vi "sandbox.vi"() -> ()   [LabVIEW 2016]
panel:
  out "Array":i32[](array[numeric])
  out "RESET":bool
  out "ADDR (7bit)":u8
  out "R (U8)":u8
  out "G (U8)":u8
  out "B (U8)":u8
  in  "RESET":bool
  in  "ADDR (7bit)":u8
  in  "B (U8)":u8
  in  "G (U8)":u8
  out "Packet":u32=8 format="%032b"
  in  "R (U8)":u8
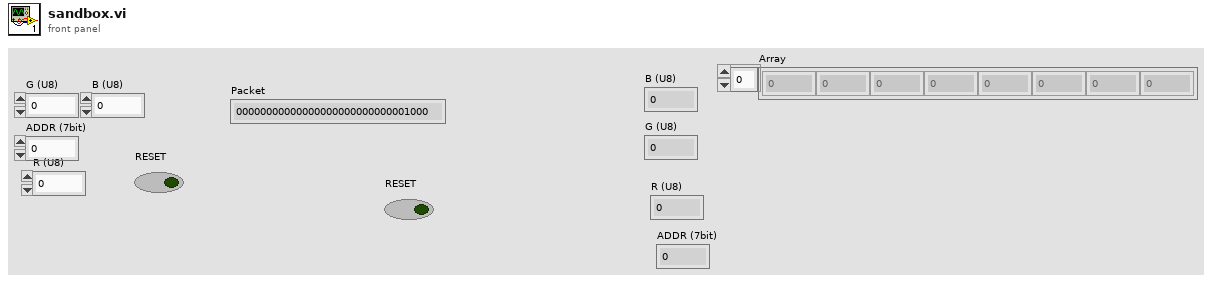
[diagram p1: front panel]
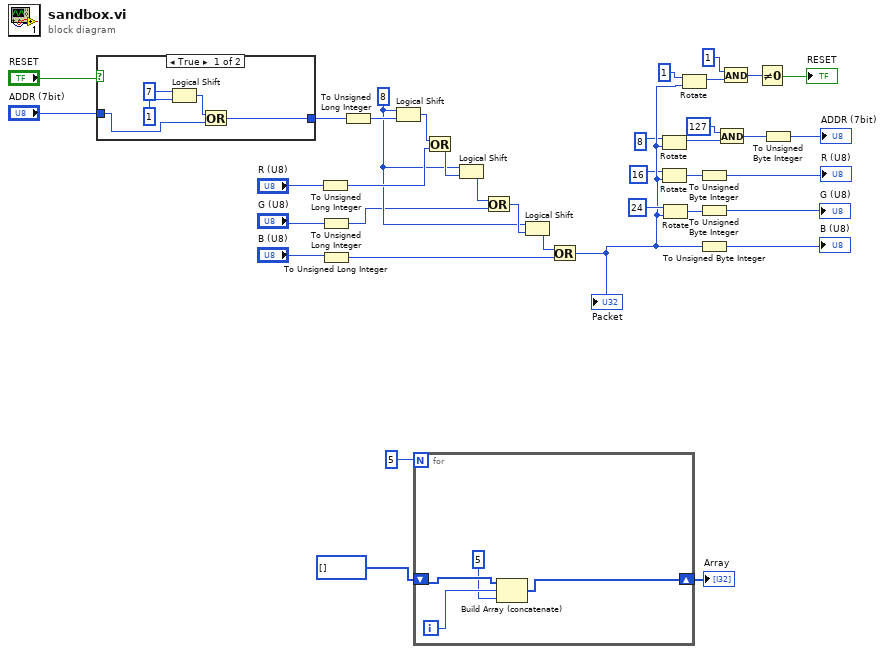
[diagram p0: block diagram]
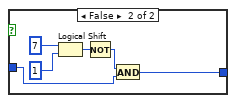
[diagram p2: hidden frame]
diagram:
  w26 = u8 8 ("x")
  n1 = case shown="True" "RESET" {
    tunnel: "ADDR (7bit)" -> [w39 w46]
    tunnel: [w38 w45] -> w33
    frame True {
      n2 = Logical Shift(y=u32 7, x=u8 1) -> (x << y=w40:u8)
      n3 = Or(x=w40, y=w39) -> (x .or. y?=w38:u8)
    }
    frame False {
      n4 = Logical Shift(y=u32 7, x=u8 1) -> (x << y=w47:u8)
      n5 = Not(x=w47) -> (.not. x?=w43:u8)
      n6 = And(x=w43, y=w46) -> (x .and. y?=w45:u8)
    }
  }
  n7 = To Unsigned Long Integer(number="R (U8)") -> (unsigned 32bit integer=w30:u32)
  n8 = To Unsigned Long Integer(number="G (U8)") -> (unsigned 32bit integer=w24:u32)
  n9 = To Unsigned Long Integer(number="B (U8)") -> (unsigned 32bit integer=w22:u32)
  n10 = To Unsigned Long Integer(number=w33) -> (unsigned 32bit integer=w32:u32)
  n11 = Logical Shift(y=w26, x=w32) -> (x << y=w31:u32)
  n12 = for {
    N: 5 ("Numeric") -> [_]
    shift-right: [w49] -> w2
    shift-left: i32[] [] -> [w52]
    i -> [w51]
    n13 = Build Array (concatenate)(w52, w51, 5) -> (w49:i32[])
  }
  "Array" <- w2
  n14 = Or(x=w31, y=w30) -> (x .or. y?=w29:u32)
  n15 = Logical Shift(y=w26, x=w29) -> (x << y=w28:u32)
  n16 = Or(x=w28, y=w24) -> (x .or. y?=w27:u32)
  n17 = Logical Shift(y=w26, x=w27) -> (x << y=w25:u32)
  n18 = Or(x=w25, y=w22) -> (x .or. y?=w16:u32)
  "Packet" <- w16
  n19 = Rotate(1:w16, 2:i16 8 ("y")) -> (0:w19:u32)
  n20 = Rotate(1:w16, 2:i16 16 ("y")) -> (0:w15:u32)
  n21 = Rotate(1:w16, 2:i16 24 ("y")) -> (0:w14:u32)
  n22 = Rotate(1:w16, 2:u32 1 ("x")) -> (0:w7:u32)
  n23 = To Unsigned Byte Integer(number=w15) -> (unsigned 8bit integer=→"R (U8)":u8)
  n24 = To Unsigned Byte Integer(number=w14) -> (unsigned 8bit integer=→"G (U8)":u8)
  n25 = To Unsigned Byte Integer(number=w16) -> (unsigned 8bit integer=→"B (U8)":u8)
  n26 = And(x=u32 127, y=w19) -> (x .and. y?=w11:u32)
  n27 = And(x=u32 1, y=w7) -> (x .and. y?=w6:u32)
  n28 = Not Equal To 0?(x=w6) -> (x != 0?=→"RESET":bool)
  n29 = To Unsigned Byte Integer(number=w11) -> (unsigned 8bit integer=→"ADDR (7bit)":u8)
